vi "intialize picoscope trigger settings.vi"(11 "PicoscopeV2 in":refnum<class "PicoscopeV2.lvclass">) -> (3 "PicoscopeV2 out":refnum<class "PicoscopeV2.lvclass">)   [LabVIEW 2020, in "PicoscopeV2.lvclass"]
uses:
  PicoscopeV2.lvclass
  PicoscopeV2.lvclass/PicoscopeV2.ctl
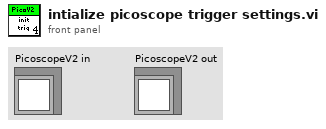
[diagram p1: front panel]
types:
  T1 = typedef "OnOffTypeDef.ctl" = enum16{"off", "on"}
  T2 = enum16{"Channel 1", "Channel 2", "Channel 3", "Channel 4", "External"}
  T3 = enum16{"Channel A", "Channel B", "Channel C", "Channel D", "Ext."}
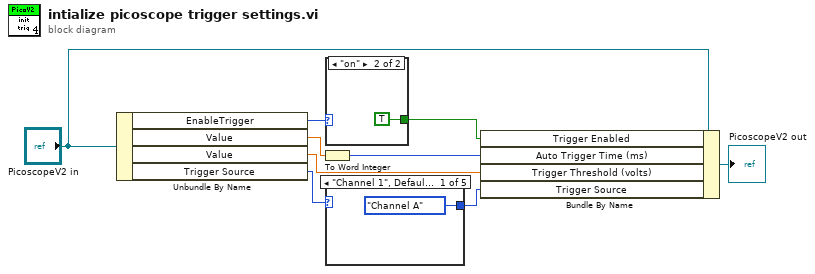
[diagram p0: block diagram]
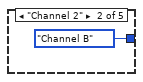
[diagram p2: hidden frame]
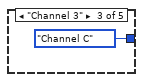
[diagram p3: hidden frame]
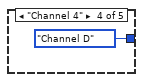
[diagram p4: hidden frame]
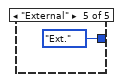
[diagram p5: hidden frame]
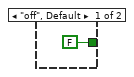
[diagram p6: hidden frame]
diagram:
  n1 = Unbundle By Name("PicoscopeV2 in") -> ("EnableTrigger"=w6:T1, "Value"=w8:dbl, "Value"=w2:dbl, "Trigger Source"=w3:T2)
  n2 = To Word Integer(number=w8) -> (16bit integer=w9:i16)
  n3 = case shown="\"on\"" w6 {
    tunnel: [FALSE TRUE] -> w7
    frame "off", Default {
    }
    frame "on" {
    }
  }
  n4 = case shown="\"Channel 1\", Default" w3 {
    tunnel: [T3."Channel A" ("Trigger Settings.Trigger Source") T3."Channel B" ("Trigger Settings.Trigger Source") T3."Channel C" ("Trigger Settings.Trigger Source") T3."Channel D" ("Trigger Settings.Trigger Source") T3."Ext." ("Trigger Settings.Trigger Source")] -> w1
    frame "Channel 1", Default {
    }
    frame "Channel 2" {
    }
    frame "Channel 3" {
    }
    frame "Channel 4" {
    }
    frame "External" {
    }
  }
  n5 = Bundle By Name(cluster="PicoscopeV2 in", "Trigger Enabled"=w7, "Auto Trigger Time (ms)"=w9, "Trigger Threshold (volts)"=w2, "Trigger Source"=w1) -> (→"PicoscopeV2 out":refnum<class "PicoscopeV2.lvclass">)
